vi "SendStatus.vi"(0 "StatusUsrEvn":T1, 2 "error in":errorcluster, 12 "Text":string) -> (22 "error out":errorcluster)   [LabVIEW 2020, in "CameraTesting.lvlib" / "CameraTesting.lvclass"]
uses:
  CameraTesting.lvclass
  ICameraTesting/ICameraTesting/TypeDef/StatusUpdated.ctl
  ICameraTesting/ICameraTesting/TypeDef/StatusRecord.ctl
  CameraTesting.lvclass/CameraTesting.ctl
  ICameraTesting/ICameraTesting/ICameraTesting.lvclass
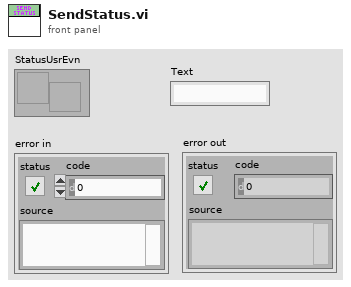
[diagram p1: front panel]
types:
  T1 = typedef "ICameraTesting.lvlib/ICameraTesting.lvclass/StatusUpdated.ctl" = refnum<user-event>
  T2 = typedef "ICameraTesting.lvlib/ICameraTesting.lvclass/StatusRecord.ctl" = cluster{"Time Stamp":timestamp, "Text":string, "Error":errorcluster}
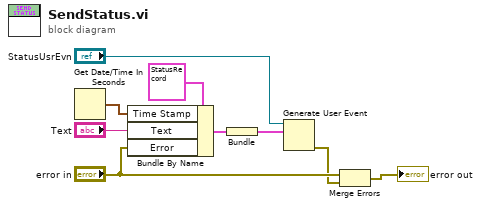
[diagram p0: block diagram]
diagram:
  n1 = Get Date/Time In Seconds() -> (seconds since 1Jan1904=w9:timestamp)
  n2 = Bundle By Name(cluster=T2 {"Time Stamp"=timestamp(0 s since 1904-01-01), "Text"="", "Error"={"status"=FALSE, "code"=0, "source"=""}} ("event data"), "Time Stamp"=w9, "Text"="Text", "Error"="error in") -> (w2:T2)
  n3 = Bundle("event data"=w2) -> (w1:cluster{"event data":T2})  [unwired: 1 in]
  n4 = Generate User Event(user event="StatusUsrEvn", event data cluster=w1) -> (error out=w4:errorcluster)  [unwired: 2 in, 1 out]
  n5 = Merge Errors("error in", w4) -> (→"error out":errorcluster)
